vi "CO2_Read.vi"() -> ()   [LabVIEW 2019]
uses:
  <vilib>/Instr/_visa.llb/VISA Configure Serial Port (Instr).vi
panel:
  out "h":dbl
  out "t":dbl
  out "c":dbl
  out "read buffer":string
  in  "VISA resource name":refnum<visa-resource-name>
  in  "stop":bool
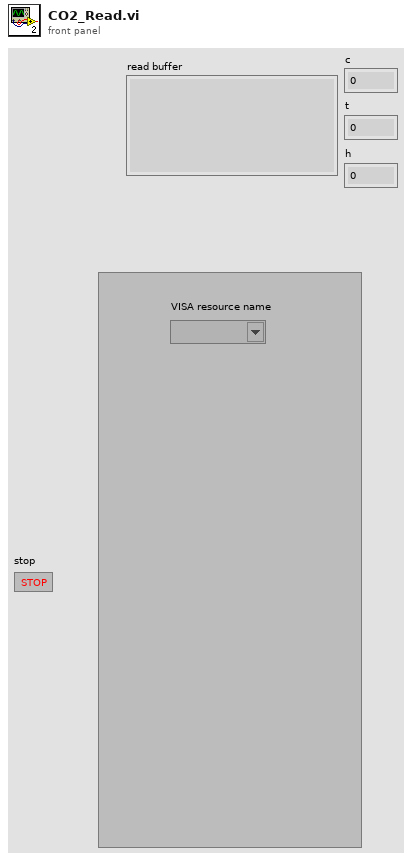
[diagram p1: front panel]
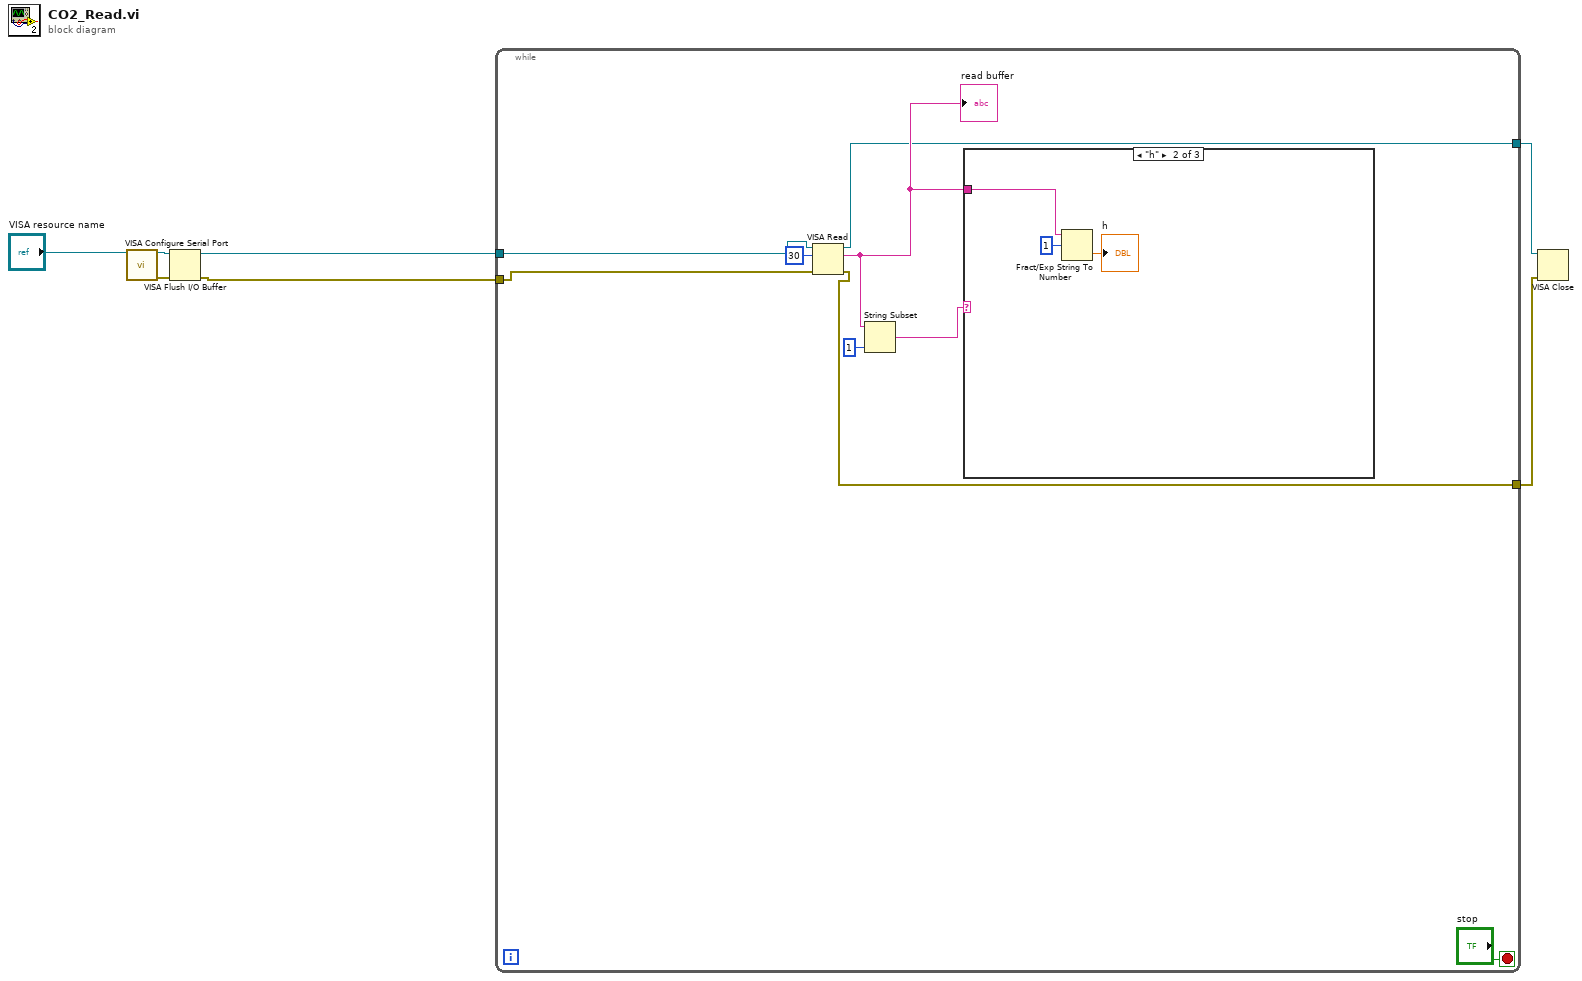
[diagram p0: block diagram]
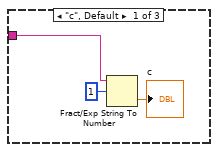
[diagram p2: hidden frame]
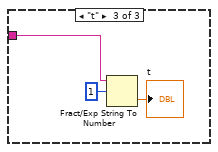
[diagram p3: hidden frame]
diagram:
  n1 = call-poly "VISA Configure Serial Port"("VISA resource name"="VISA resource name") -> ("VISA resource name out"=w4:refnum<visa-resource-name>, "error out"=w5:errorcluster)  [unwired: 13 in]
  n2 = VISA Flush I/O Buffer(VISA resource name=w4, error in (no error)=w5) -> (VISA resource name out=w6:refnum<visa-resource-name>, error out=w3:errorcluster)  [unwired: 1 in]
  n3 = while {
    tunnel: w6 -> [w13]
    tunnel: w3 -> [w14]
    tunnel: [w9] -> w2
    tunnel: [w8] -> w1
    stop <- "stop" stop-if-true
    n4 = VISA Read(VISA resource name=w13, byte count=u32 30, error in (no error)=w14) -> (VISA resource name out=w9:refnum<visa-resource-name>, read buffer=w10:string, error out=w8:errorcluster)  [unwired: 1 out]
    "read buffer" <- w10
    n5 = String Subset(string=w10, length (rest)=1 ("length (rest)")) -> (substring=w12:string)  [unwired: 1 in]
    n6 = case shown="\"h\"" w12 {
      tunnel: w10 -> [w18 w21 w24]
      frame "c", Default {
        n7 = Fract/Exp String To Number(string=w18, offset=1) -> (number=→"c":dbl)  [unwired: 2 in, 1 out]
      }
      frame "h" {
        n8 = Fract/Exp String To Number(string=w21, offset=1) -> (number=→"h":dbl)  [unwired: 2 in, 1 out]
      }
      frame "t" {
        n9 = Fract/Exp String To Number(string=w24, offset=1) -> (number=→"t":dbl)  [unwired: 2 in, 1 out]
      }
    }
  }
  n10 = VISA Close(VISA resource name=w2, error in (no error)=w1) -> ()  [unwired: 1 out]
